vi "Progress Bar Popup.vi"(7 "Abort visible? (T)":bool, 9 "Message (Please Wait...)":string="Please Wait...", 10 "Current Iteration":u32, 11 "Total Iterations":u32) -> (1 "Aborted":bool)   [LabVIEW 2014]
uses:
  <vilib>/Utility/miscctls.llb/LVPointTypeDef.ctl
panel:
  in  "Abort Button":bool
  out "String":string
  out "Slide":u8(slide) scale=0.0..100.0
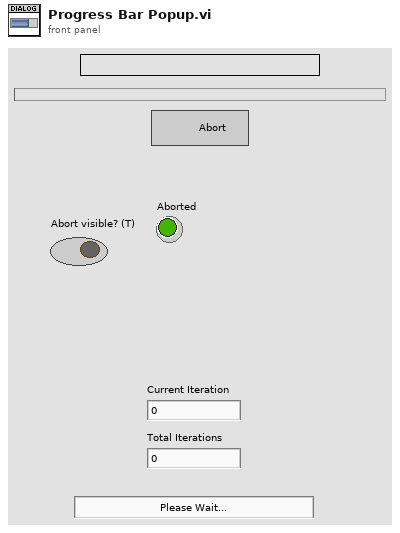
[diagram p1: front panel]
types:
  T1 = typedef "LVPointTypeDef.ctl" = cluster{"Horizontal":i16, "Vertical":i16}
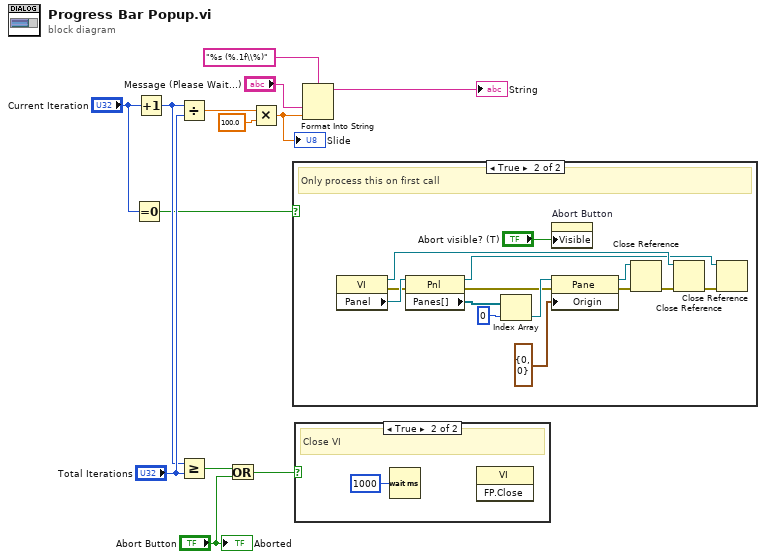
[diagram p0: block diagram]
diagram:
  n1 = Equal To 0?(x="Current Iteration") -> (x = 0?=w4:bool)
  n2 = Increment(x="Current Iteration") -> (x+1=w8:u32)
  n3 = Divide(x=w8, y="Total Iterations") -> (x/y=w13:dbl)
  n4 = Greater Or Equal?(x=w8, y="Total Iterations") -> (x >= y?=w9:bool)
  n5 = Or(x=w9, y="Abort Button") -> (x .or. y?=w7:bool)
  n6 = Multiply(x=w13, y=100.0) -> (x*y=w11:dbl)
  "Slide" <- w11
  n7 = case shown="True" w4 {
    frame False {
      # "Not first call."
    }
    frame True {
      # "Only process this on first call"
      n8 = property class="VI"() -> (reference out=w17:refnum<vi>, error out=w21:errorcluster, "Panel"=w23:refnum<vi>)  [unwired: 2 in]
      n9 = property class="Pnl"(reference=w23, error in=w21) -> (reference out=w15:refnum<vi>, error out=w20:errorcluster, "Panes[]"=w24:refnum<vi>[])
      n10 = Index Array(array=w24, index=0) -> (element=w26:refnum<vi>)
      n11 = property on="Abort Button" class="Bool"("Visible"="Abort visible? (T)") -> ()  [unwired: 2 in, 2 out]
      n12 = property class="Pane"(reference=w26, error in=w20, "Origin"=T1 {"Horizontal"=0, "Vertical"=0}) -> (reference out=w22:refnum<vi>, error out=w19:errorcluster)
      n13 = Close Reference(reference=w22, error in (no error)=w19) -> (error out=w18:errorcluster)
      n14 = Close Reference(reference=w17, error in (no error)=w18) -> (error out=w16:errorcluster)
      n15 = Close Reference(reference=w15, error in (no error)=w16) -> ()  [unwired: 1 out]
    }
  }
  n16 = case shown="True" w7 {
    frame False {
      # "Don't close"
    }
    frame True {
      # "Close VI"
      n17 = Wait (ms)(milliseconds to wait=u32 1000) -> ()  [unwired: 1 out]
      n18 = invoke class="VI" method="FP.Close"() -> ()  [unwired: 3 in, 3 out]
    }
  }
  n19 = Format Into String(format string="%s (%.1f\\%)", "Message (Please Wait...)", w11) -> (resulting string=→"String":string)  [unwired: 2 in, 1 out]
  "Aborted" <- "Abort Button"
